vi "CheckArgsInRange.vi"(4 "ReadLength (bytes)":u8, 5 "Address":u16=16384 caption="Address [16384=Unadressed]" max=16384, 6 "Register":i32, 9 "Argument":i32, 10 "CommandDescriptor in":T1) -> (2 "In Range?":bool, 3 "Not Group/Global?":bool)   [LabVIEW 2021]
uses:
  PololuCommandDescriptor.ctl
  TicCommandType.ctl
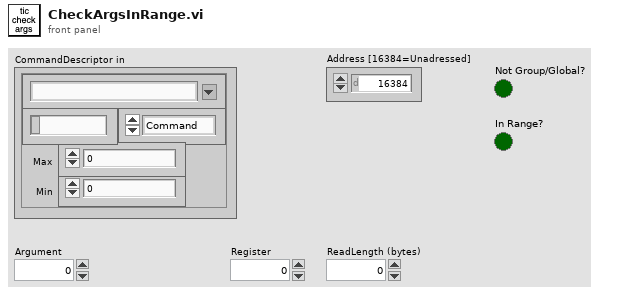
[diagram p1: front panel]
types:
  T1 = typedef "PololuCommandDescriptor.ctl" = cluster{"PololuCommand":string, "Mnemonic":string, "CommandType":T2, "Min":i32, "Max":i32}
  T2 = typedef "TicCommandType.ctl" = enum16{"Command", "7-bitWrite", "32-bitWrite", "BlockRead"}
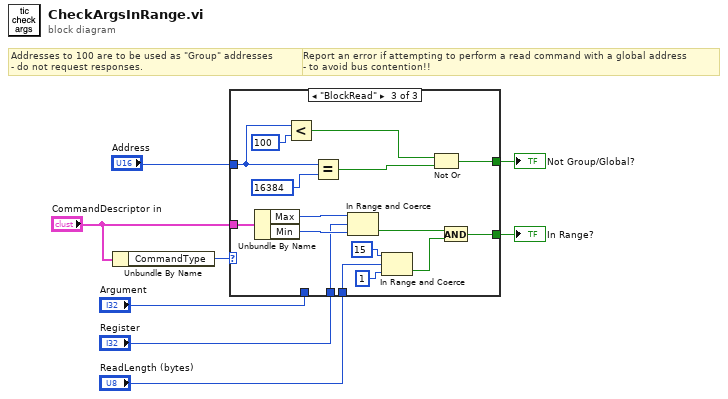
[diagram p0: block diagram]
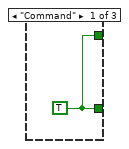
[diagram p2: hidden frame]
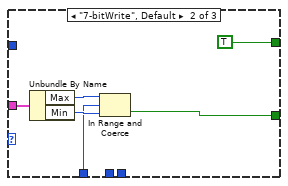
[diagram p3: hidden frame]
diagram:
  # "Addresses to 100 are to be used as \"Group\" addresses\n- do not request responses."
  # "Report an error if attempting to perform a read command with a global address\n- to avoid bus contention!!"
  n1 = Unbundle By Name("CommandDescriptor in") -> ("CommandType"=w5:T2)
  n2 = case shown="\"BlockRead\"" w5 {
    tunnel: "CommandDescriptor in" -> [_ w13 w28]
    tunnel: "Register" -> [_ _ w29]
    tunnel: [w9 w12 w24] -> w7
    tunnel: "ReadLength (bytes)" -> [_ _ w27]
    tunnel: "Argument" -> [_ w11 _]
    tunnel: "Address" -> [_ _ w20]
    tunnel: [w9 TRUE w16] -> w1
    frame "Command" {
      w9 = TRUE
    }
    frame "7-bitWrite", Default {
      n3 = Unbundle By Name(w13) -> ("Max"=w15:i32, "Min"=w14:i32)
      n4 = In Range and Coerce(upper limit=w15, x=w11, lower limit=w14) -> (In Range?=w12:bool)  [unwired: 1 out]
    }
    frame "BlockRead" {
      n5 = Unbundle By Name(w28) -> ("Max"=w31:i32, "Min"=w30:i32)
      n6 = Less?(x=w20, y=u16 100) -> (x < y?=w18:bool)
      n7 = Equal?(x=w20, y=u16 16384) -> (x = y?=w17:bool)
      n8 = In Range and Coerce(upper limit=w31, x=w29, lower limit=w30) -> (In Range?=w23:bool)  [unwired: 1 out]
      n9 = In Range and Coerce(upper limit=u8 15, x=w27, lower limit=u8 1) -> (In Range?=w22:bool)  [unwired: 1 out]
      n10 = Not Or(1:w17, 2:w18) -> (0:w16:bool)
      n11 = And(x=w23, y=w22) -> (x .and. y?=w24:bool)
    }
  }
  "In Range?" <- w7
  "Not Group/Global?" <- w1
